vi "Agilent Read Scanlist.vi"(2 "error in (no error)":errorcluster, 3 "VISA Resource Name":refnum<visa-resource-name>) -> (0 "error out":errorcluster, 1 "Output Data (Numbers Only)":dbl[](array[numeric]))   [LabVIEW 2012]
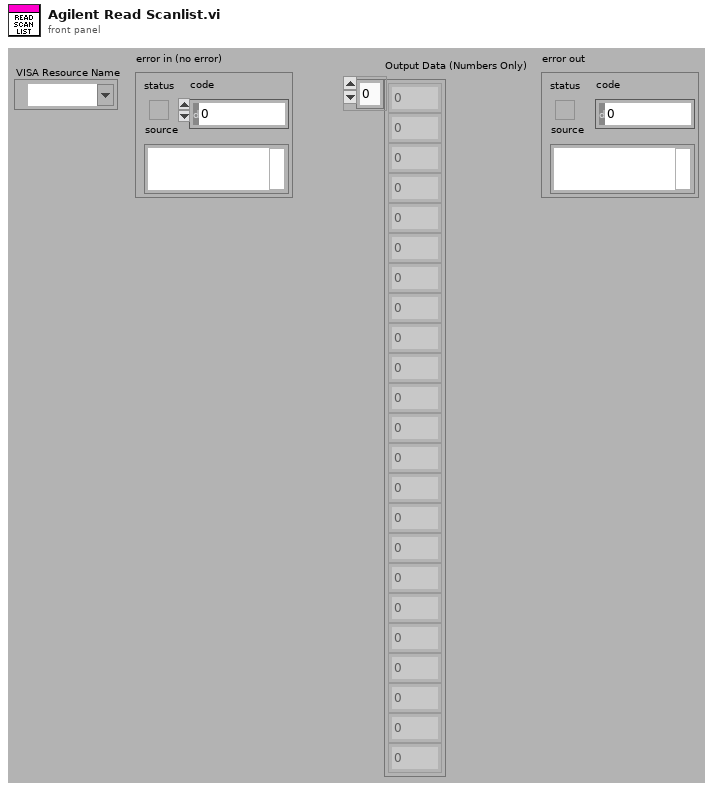
[diagram p1: front panel]
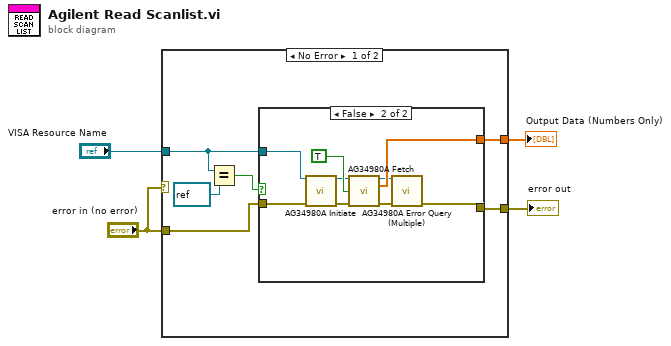
[diagram p0: block diagram]
diagram:
  n1 = case shown="No Error" "error in (no error)" {
    selector: "error in (no error)" -> [_ w21]
    tunnel: [w10 w21] -> w4
    tunnel: "error in (no error)" -> [w9 _]
    tunnel: [w8 _] -> w3
    tunnel: "VISA Resource Name" -> [w6 _]
    frame No Error {
      n2 = Equal?(x=w6, y=refnum<visa-resource-name> refnum ("VISA Resource Name 2")) -> (x = y?=w5:bool)
      n3 = case shown="False" w5 {
        tunnel: [w11 w20] -> w10
        tunnel: w9 -> [w11 w19]
        tunnel: [_ w18] -> w8
        tunnel: w6 -> [_ w17]
        frame True {
        }
        frame False {
          n4 = call "AG34980A Initiate.vi"("VISA resource name"=w17, "error in (no error)"=w19) -> ("VISA resource name out"=w14:refnum<visa-resource-name>, "error out"=w12:errorcluster)  [unwired: 12 in]
          n5 = call "AG34980A Fetch.vi"("VISA resource name"=w14, "Numbers Only (T:On)"=TRUE, "error in (no error)"=w12) -> ("VISA resource name out"=w15:refnum<visa-resource-name>, "Output Data (Numbers Only)"=w18:dbl[], "error out"=w13:errorcluster)  [unwired: 8 in, 2 out]
          n6 = call "AG34980A Error Query (Multiple).vi"("VISA resource name"=w15, "error in (no error)"=w13) -> ("error out"=w20:errorcluster)  [unwired: 10 in, 3 out]
        }
      }
    }
    frame Error {
    }
  }
  "error out" <- w4
  "Output Data (Numbers Only)" <- w3
